vi "Current Limit.vi"(9 "Robot Max Current":dbl, 10 "Current Right":dbl format="%#_13g", 11 "Current Left":dbl format="%#_13g") -> (1 "Max Voltage Right":dbl format="%#_13g", 2 "Max Voltage left":dbl format="%#_13g", 3 "Total current":dbl)   [LabVIEW 2015]
uses:
  <vilib>/express/express arith-compare/Formula/XNode/ExpressFormulaBlockNode.xnode
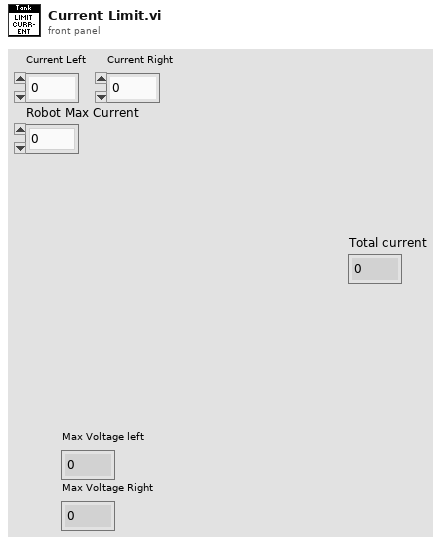
[diagram p1: front panel]
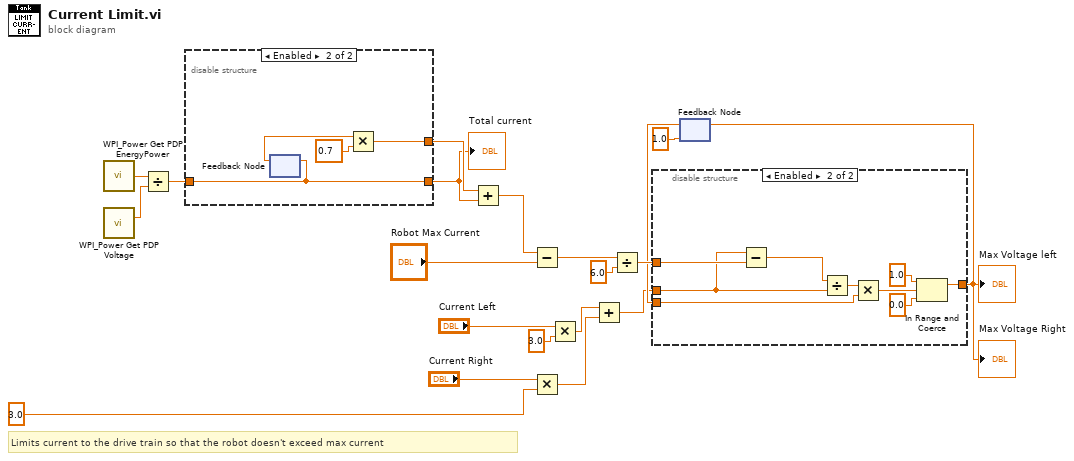
[diagram p0: block diagram]
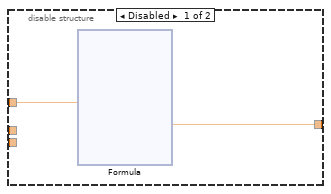
[diagram p2: hidden frame]
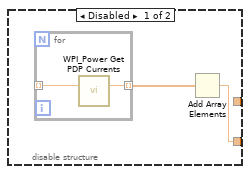
[diagram p3: hidden frame]
diagram:
  # "Limits current to the drive train so that the robot doesn't exceed max current"
  n1 = call <vilib>:"WPI_Power Get PDP EnergyPower.vi"() -> ("Power (W)"=w10:dbl)  [unwired: 13 in, 2 out]
  n2 = call <vilib>:"WPI_Power Get PDP Voltage.vi"() -> ("voltage (V)"=w14:dbl)  [unwired: 14 in, 1 out]
  n3 = Divide(x=w10, y=w14) -> (x/y=w9:dbl)
  n4 = disable-structure shown="Enabled" {
    disable-tunnel: [w23 w26] -> w11
    disable-tunnel: [_ w27] -> w12
    disable-tunnel: w9 -> [_ w26]
    frame Disabled {
      n5 = for {
        tunnel: [w24] -> w22 mode=indexing
        tunnel: [w25] -> w21 mode=indexing
        n6 = call <vilib>:"WPI_Power Get PDP Currents.vi"("PDP Channel"=w24) -> ("current (A)"=w25:dbl)  [unwired: 12 in, 2 out]
      }
      n7 = Add Array Elements(numeric array=w21) -> (sum=w23:dbl)
    }
    frame Enabled {
      n8 = feedback-in #1(w26) -> ()
      n9 = feedback #1() -> (w28:dbl)  [unwired: 1 in]
      n10 = Multiply(x=w28, y=0.7) -> (x*y=w27:dbl)
    }
  }
  "Total current" <- w11
  n11 = Add(x=w12, y=w11) -> (x+y=w13:dbl)
  n12 = Subtract(x=w13, y="Robot Max Current") -> (x-y=w17:dbl)
  n13 = Multiply(x="Current Right", y=3.0) -> (x*y=w3:dbl)
  n14 = Multiply(x="Current Left", y=3.0) -> (x*y=w4:dbl)
  n15 = Add(x=w4, y=w3) -> (x+y=w2:dbl)
  n16 = Divide(x=w17, y=6.0) -> (x/y=w19:dbl)
  n17 = feedback #2(1.0) -> (w16:dbl)
  n18 = disable-structure shown="Enabled" {
    disable-tunnel: [w31 w45] -> w15
    disable-tunnel: w19 -> [w30 w51]
    disable-tunnel: w2 -> [_ w43]
    disable-tunnel: w16 -> [_ w49]
    frame Disabled {
      n19 = xnode "Formula"("X"=w30) -> ("Result"=w31:dbl, "p"=w32:dbl)  [unwired: 1 in, 1 out]
    }
    frame Enabled {
      n20 = Subtract(x=w43, y=w51) -> (x-y=w44:dbl)
      n21 = Divide(x=w44, y=w43) -> (x/y=w50:dbl)
      n22 = Multiply(x=w50, y=w49) -> (x*y=w48:dbl)
      n23 = In Range and Coerce(upper limit=1.0, x=w48, lower limit=0.0) -> (coerced(x)=w45:dbl)  [unwired: 1 out]
    }
  }
  "Max Voltage left" <- w15
  "Max Voltage Right" <- w15
  n24 = feedback-in #2(w15) -> ()
